vi "GetTextFromNode.vi"(8 "error in (no error)":errorcluster, 9 "Failure db-folderpath":string, 10 "node in":refnum<k20>, 11 "Text":string) -> (0 "error out":errorcluster, 2 "node out":refnum<k20>, 3 "Failure-db path":string)   [LabVIEW 2011]
uses:
  <vilib>/xml/NI_XML.lvlib
  Program Files (x86)/National Instruments/LabVIEW 2011/resource/objmgr/DOMUserDefRef.rc
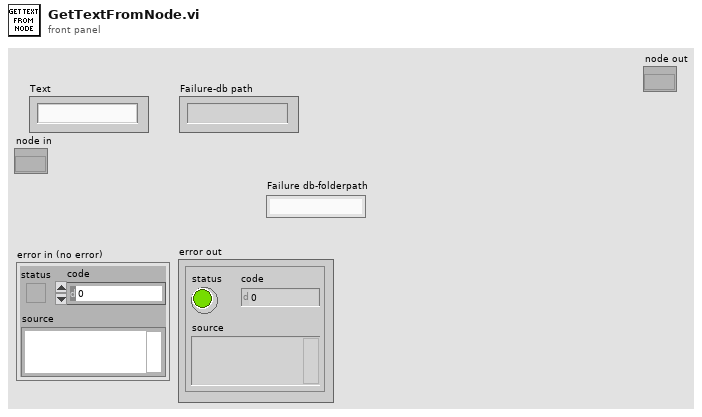
[diagram p1: front panel]
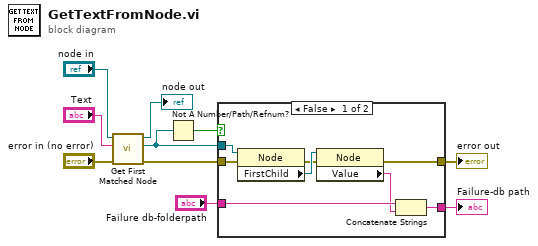
[diagram p0: block diagram]
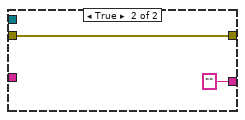
[diagram p2: hidden frame]
diagram:
  n1 = call <vilib>:"Get First Matched Node.vi"("error in (no error)"="error in (no error)", "XPath expression"="Text", "node in"="node in") -> ("error out"=w5:errorcluster, "node result"=w9:refnum<k20>, "node out"=→"node out":refnum<k20>)  [unwired: 6 in]
  n2 = Not A Number/Path/Refnum?(number/path/refnum=w9) -> (NaN/Path/Refnum?=w8:bool)
  n3 = case shown="False" w8 {
    tunnel: w9 -> [w18 _]
    tunnel: [w11 "" ("Value")] -> w10
    tunnel: w5 -> [w16 w19]
    tunnel: [w14 w19] -> w4
    tunnel: "Failure db-folderpath" -> [w13 _]
    frame False {
      n4 = property class="Node"(reference=w18, error in=w16) -> (error out=w15:errorcluster, "FirstChild"=w17:refnum<k20>)  [unwired: 1 out]
      n5 = property class="Node"(reference=w17, error in=w15) -> (error out=w14:errorcluster, "Value"=w12:string)  [unwired: 1 out]
      n6 = Concatenate Strings(w13, w12) -> (w11:string)
    }
    frame True {
    }
  }
  "Failure-db path" <- w10
  "error out" <- w4
